vi "MapChannels.vi"(8 "error in (no error)":errorcluster caption="错误输入（无错误）", 11 "XYPlot 输入":refnum<class "XYPlot.lvclass">) -> (0 "error out":errorcluster caption="错误输出", 3 "XYPlot 输出":refnum<class "XYPlot.lvclass">)   [LabVIEW 2018, in "DataDisplay.lvlib" / "XYPlot.lvclass"]
uses:
  XYPlot.lvclass
  XYPlot.lvclass/XYPlot.ctl
  TypeDefine/DD_Command.ctl
  DataDisplay.lvlib
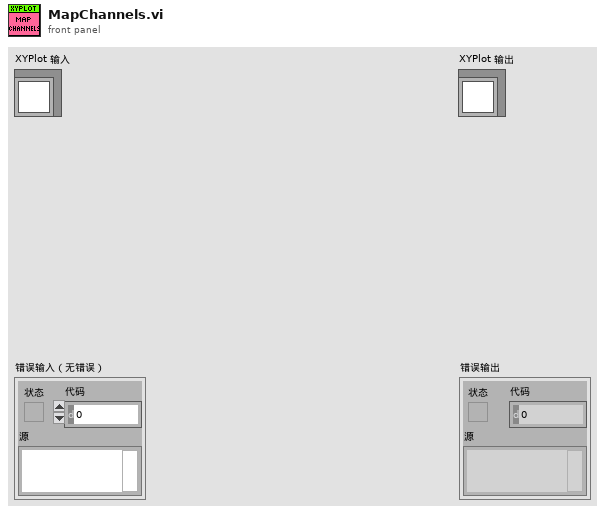
[diagram p1: front panel]
types:
  T1 = typedef "DataDisplay.lvlib/DD_Command.ctl" = cluster{"消息":string, "参数":variant}
  T2 = typedef "DataDisplay.lvlib/DD_CommandQ.ctl" = refnum<queue>
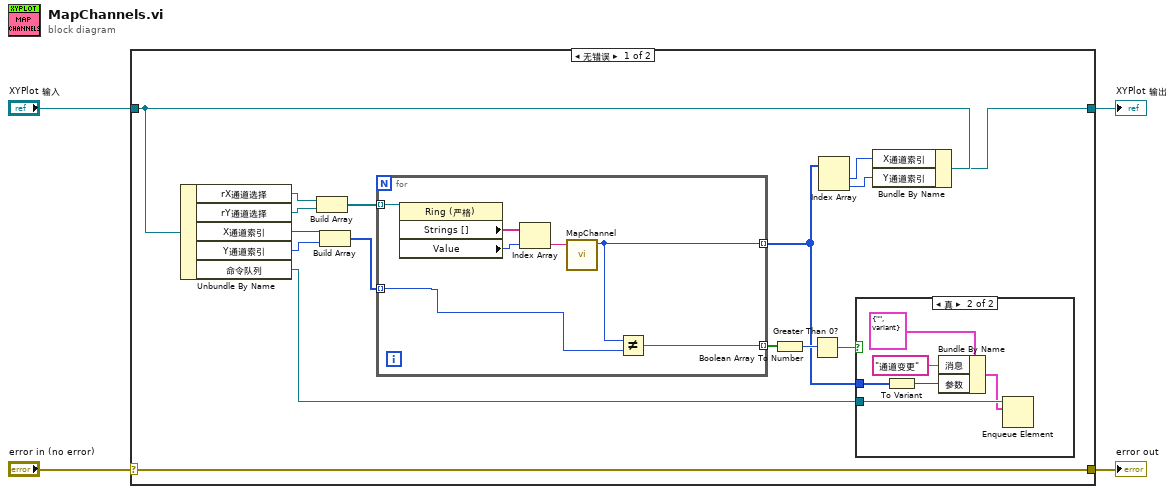
[diagram p0: block diagram]
diagram:
  n1 = case shown="无错误" "error in (no error)" {
    selector: "error in (no error)" -> [w20 w35]
    tunnel: [w20 w35] -> w3
    tunnel: [w9 w34] -> w1
    tunnel: "XYPlot 输入" -> [w19 w34]
    frame No Error {
      n2 = Unbundle By Name(w19) -> ("rX通道选择"=w18:refnum<vi>, "rY通道选择"=w17:refnum<vi>, "X通道索引"=w12:i32, "Y通道索引"=w11:i32, "命令队列"=w6:T2)
      n3 = Build Array(w18, w17) -> (w16:refnum<vi>[])
      n4 = Build Array(w12, w11) -> (w10:i32[])
      n5 = for {
        tunnel: w16 -> [w33] mode=indexing
        tunnel: w10 -> [w28] mode=indexing
        tunnel: [w29] -> w15 mode=indexing
        tunnel: [w27] -> w5 mode=indexing
        n6 = property class="Ring (严格)"(reference=w33) -> ("Strings []"=w32:string[], "Value"=w31:u16)  [unwired: 1 in, 2 out]
        n7 = Index Array(array=w32, index=w31) -> (element=w30:string)
        n8 = call "MapChannel.vi"("通道名称"=w30) -> ("索引"=w27:i32)  [unwired: 9 in, 1 out]
        n9 = Not Equal?(x=w27, y=w28) -> (x != y?=w29:bool)
      }
      n10 = Boolean Array To Number(Boolean array=w15) -> (number=w14:u32)
      n11 = Greater Than 0?(x=w14) -> (x > 0?=w13:bool)
      n12 = Index Array(array=w5) -> (element #1=w8:i32, element #2=w7:i32)  [unwired: 2 in]
      n13 = case shown="真" w13 {
        tunnel: w6 -> [_ w26]
        tunnel: w5 -> [_ w21]
        frame False {
        }
        frame True {
          n14 = To Variant(anything=w21) -> (Variant=w22:variant)
          n15 = Bundle By Name(cluster=T1 {"消息"="", "参数"=variant} ("元素"), "消息"="通道变更", "参数"=w22) -> (w24:T1)
          n16 = Enqueue Element(queue=w26, element=w24) -> ()  [unwired: 2 in, 3 out]
        }
      }
      n17 = Bundle By Name(cluster=w19, "X通道索引"=w8, "Y通道索引"=w7) -> (w9:refnum<class "XYPlot.lvclass">)
    }
    frame Error {
    }
  }
  "error out" <- w3
  "XYPlot 输出" <- w1
